vi "Example_resistor_pass_fail.vi"() -> ()   [LabVIEW 2022 SP3]
uses:
  usbtmc_scpi_labtool.lvlib
panel:
  out "sample":i32
  out "result":enum16{"not mounted", "out of spec", "in spec"}(ring)
  in  "test":bool
  in  "stop":bool
  in  "VISA resource name in":refnum<visa-resource-name>
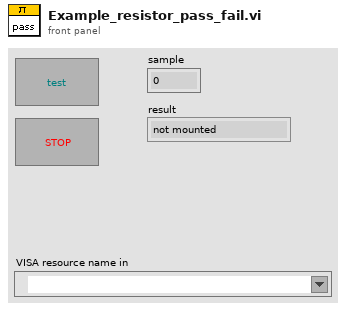
[diagram p1: front panel]
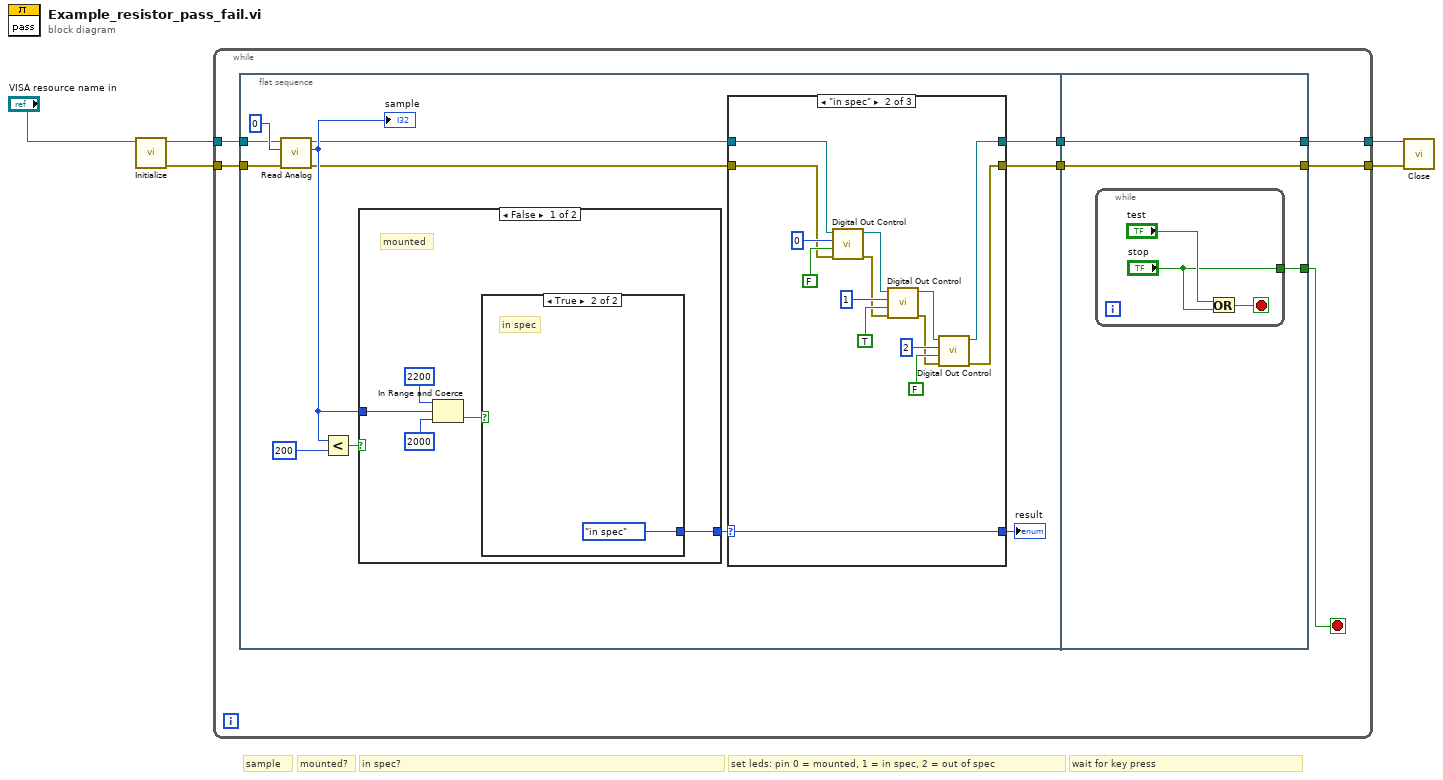
[diagram p0: block diagram]
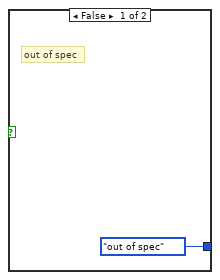
[diagram p2: hidden frame]
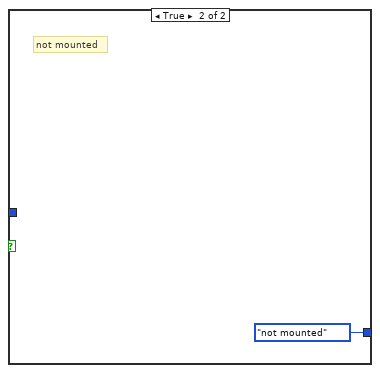
[diagram p3: hidden frame]
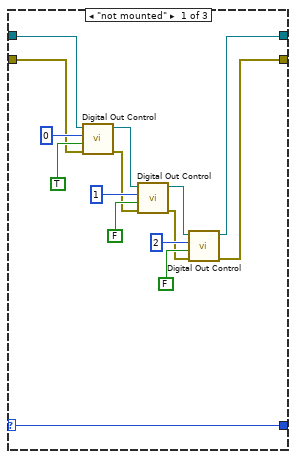
[diagram p4: hidden frame]
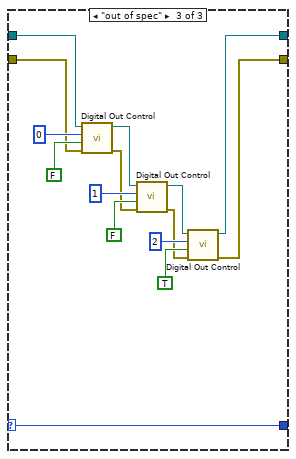
[diagram p5: hidden frame]
diagram:
  # "sample"
  # "in spec?"
  # "mounted?"
  # "set leds: pin 0 = mounted, 1 = in spec, 2 = out of spec"
  # "wait for key press"
  n1 = call "Initialize.vi"("VISA resource name in"="VISA resource name in") -> ("error out"=w3:errorcluster, "VISA resource name out"=w4:refnum<visa-resource-name>)  [unwired: 9 in]
  n2 = while {
    tunnel: w4 -> [w12]
    tunnel: w3 -> [w11]
    tunnel: [w7] -> w2
    tunnel: [w6] -> w1
    stop <- w10 stop-if-true
    n3 = flat-sequence {
      tunnel: w12 -> [w16]
      tunnel: w11 -> [w15]
      tunnel: [w14] -> w9
      tunnel: [w13] -> w8
      tunnel: [w80] -> w10
      tunnel: [w79] -> w7
      tunnel: w9 -> [w79]
      tunnel: [w78] -> w6
      tunnel: w8 -> [w78]
      frame #0 {
        n4 = call "Read Analog.vi"("error in (no error)"=w15, "Pin"=u8 0, "VISA resource name"=w16) -> ("error out"=w17:errorcluster, "analog out"=w19:i32, "VISA resource name out"=w18:refnum<visa-resource-name>)  [unwired: 6 in]
        "sample" <- w19
        n5 = Less?(x=w19, y=200) -> (x < y?=w21:bool)
        n6 = case shown="False" w21 {
          tunnel: [w25 enum16{"not mounted", "out of spec", "in spec"}."not mounted" ("Enum")] -> w20
          tunnel: w19 -> [w29 _]
          frame False {
            # "mounted"
            n7 = In Range and Coerce(upper limit=2200, x=w29, lower limit=2000) -> (In Range?=w26:bool)  [unwired: 1 out]
            n8 = case shown="True" w26 {
              tunnel: [enum16{"not mounted", "out of spec", "in spec"}."out of spec" ("Enum") enum16{"not mounted", "out of spec", "in spec"}."in spec" ("Enum")] -> w25
              frame False {
                # "out of spec"
              }
              frame True {
                # "in spec"
              }
            }
          }
          frame True {
            # "not mounted"
          }
        }
        n9 = case shown="\"in spec\"" w20 {
          selector: w20 -> [w33 w48 w77]
          tunnel: [w33 w48 w77] -> w22
          tunnel: w18 -> [w36 w56 w66]
          tunnel: w17 -> [w37 w50 w65]
          tunnel: [w35 w51 w64] -> w14
          tunnel: [w34 w49 w63] -> w13
          frame "not mounted" {
            n10 = call "Digital Out Control.vi"("VISA resource name"=w36, "Pin"=u8 0, "Enable Pin (F: Off)"=TRUE, "error in (no error)"=w37) -> ("VISA resource name out"=w41:refnum<visa-resource-name>, "error out"=w40:errorcluster)  [unwired: 5 in]
            n11 = call "Digital Out Control.vi"("VISA resource name"=w41, "Pin"=u8 1, "Enable Pin (F: Off)"=FALSE, "error in (no error)"=w40) -> ("VISA resource name out"=w38:refnum<visa-resource-name>, "error out"=w39:errorcluster)  [unwired: 5 in]
            n12 = call "Digital Out Control.vi"("VISA resource name"=w38, "Pin"=u8 2, "Enable Pin (F: Off)"=FALSE, "error in (no error)"=w39) -> ("VISA resource name out"=w35:refnum<visa-resource-name>, "error out"=w34:errorcluster)  [unwired: 5 in]
          }
          frame "in spec" {
            n13 = call "Digital Out Control.vi"("VISA resource name"=w56, "Pin"=u8 0, "Enable Pin (F: Off)"=FALSE, "error in (no error)"=w50) -> ("VISA resource name out"=w55:refnum<visa-resource-name>, "error out"=w54:errorcluster)  [unwired: 5 in]
            n14 = call "Digital Out Control.vi"("VISA resource name"=w55, "Pin"=u8 1, "Enable Pin (F: Off)"=TRUE, "error in (no error)"=w54) -> ("VISA resource name out"=w52:refnum<visa-resource-name>, "error out"=w53:errorcluster)  [unwired: 5 in]
            n15 = call "Digital Out Control.vi"("VISA resource name"=w52, "Pin"=u8 2, "Enable Pin (F: Off)"=FALSE, "error in (no error)"=w53) -> ("VISA resource name out"=w51:refnum<visa-resource-name>, "error out"=w49:errorcluster)  [unwired: 5 in]
          }
          frame "out of spec" {
            n16 = call "Digital Out Control.vi"("VISA resource name"=w66, "Pin"=u8 0, "Enable Pin (F: Off)"=FALSE, "error in (no error)"=w65) -> ("VISA resource name out"=w70:refnum<visa-resource-name>, "error out"=w69:errorcluster)  [unwired: 5 in]
            n17 = call "Digital Out Control.vi"("VISA resource name"=w70, "Pin"=u8 1, "Enable Pin (F: Off)"=FALSE, "error in (no error)"=w69) -> ("VISA resource name out"=w67:refnum<visa-resource-name>, "error out"=w68:errorcluster)  [unwired: 5 in]
            n18 = call "Digital Out Control.vi"("VISA resource name"=w67, "Pin"=u8 2, "Enable Pin (F: Off)"=TRUE, "error in (no error)"=w68) -> ("VISA resource name out"=w64:refnum<visa-resource-name>, "error out"=w63:errorcluster)  [unwired: 5 in]
          }
        }
        "result" <- w22
      }
      frame #1 {
        n19 = while {
          tunnel: ["stop"] -> w80
          stop <- w83 stop-if-true
          n20 = Or(x="test", y="stop") -> (x .or. y?=w83:bool)
        }
      }
    }
  }
  n21 = call "Close.vi"("error in (no error)"=w1, "VISA resource name"=w2) -> ()  [unwired: 10 in]
